vi "LVL device cluster to String.vi"(11 "Level Meter":T1) -> (3 "Data to send":string=":HEL:RES:ZERO:1.0:FULL:2.0:RES:PREP:MAG:3.0:TIM:4.0:PREP:PULS:MAG:5.0:TIM:6.0:DEL:7.0:PULS:HEL:NIT:FREQ:ZERO:8.0:FULL:9.0:FREQ:PPS:10.0:NIT")   [LabVIEW 2019, in "Mercury iXX.lvlib" / "Level Meter.lvlib"]
uses:
  Level Meter.lvlib
  Controls/Level Meter (Set).ctl
  Controls/Helium Configuration.ctl
  Controls/Resistance Configuration.ctl
  Controls/Pre-Pulse.ctl
  Controls/Pulse.ctl
  Controls/Nitrogen Configuration.ctl
  Controls/Frequency Configuration.ctl
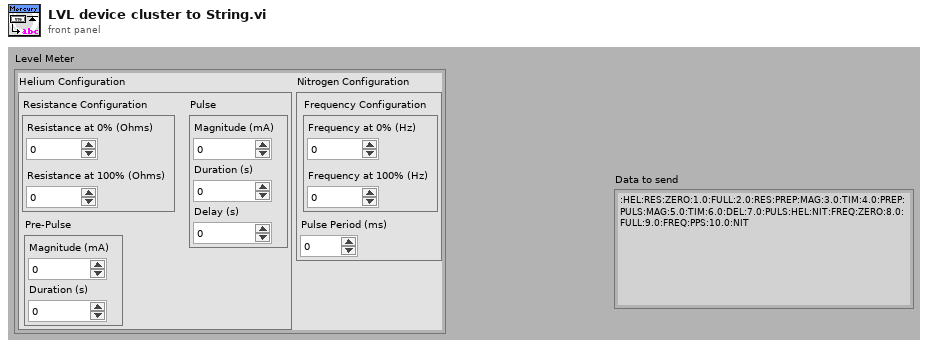
[diagram p1: front panel]
types:
  T1 = typedef "Mercury iXX.lvlib/Level Meter.lvlib/Level Meter (Set).ctl" = cluster{"Helium Configuration":T2, "Nitrogen Configuration":T6}
  T2 = typedef "Mercury iXX.lvlib/Level Meter.lvlib/Helium Configuration.ctl" = cluster{"Resistance Configuration":T3, "Pre-Pulse":T4, "Pulse":T5}
  T3 = typedef "Mercury iXX.lvlib/Level Meter.lvlib/Resistance Configuration.ctl" = cluster{"Res 0%":dbl, "Res 100%":dbl}
  T4 = typedef "Mercury iXX.lvlib/Level Meter.lvlib/Pre-Pulse.ctl" = cluster{"Magnitude":dbl, "Duration":dbl}
  T5 = typedef "Mercury iXX.lvlib/Level Meter.lvlib/Pulse.ctl" = cluster{"Magnitude":dbl, "Duration":dbl, "Delay":dbl}
  T6 = typedef "Mercury iXX.lvlib/Level Meter.lvlib/Nitrogen Configuration.ctl" = cluster{"Frequency Configuration":T7, "Pulse Period":dbl}
  T7 = typedef "Mercury iXX.lvlib/Level Meter.lvlib/Frequency Configuration.ctl" = cluster{"Freq 0%":dbl, "Freq 100%":dbl}
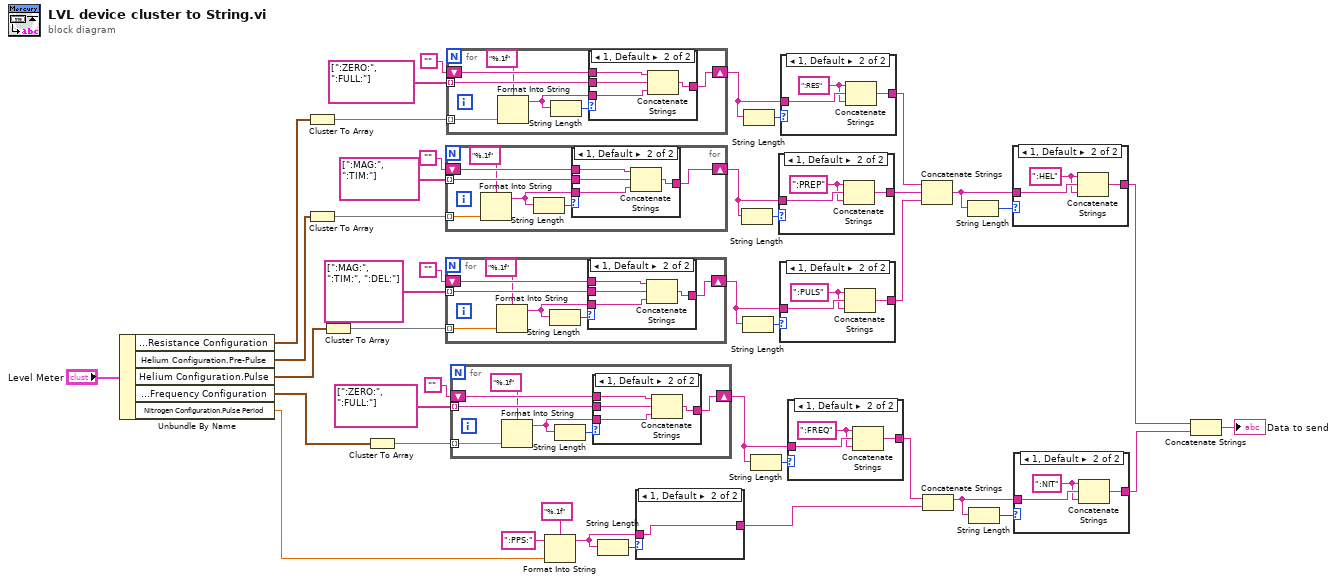
[diagram p0: block diagram]
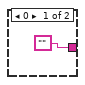
[diagram p2: hidden frame]
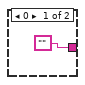
[diagram p3: hidden frame]
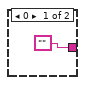
[diagram p4: hidden frame]
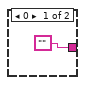
[diagram p5: hidden frame]
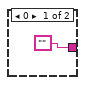
[diagram p6: hidden frame]
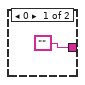
[diagram p7: hidden frame]
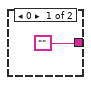
[diagram p10: hidden frame]
diagram:
  n1 = Unbundle By Name("Level Meter") -> ("Helium Configuration.Resistance Configuration"=w39:T3, "Helium Configuration.Pre-Pulse"=w34:T4, "Helium Configuration.Pulse"=w33:T5, "Nitrogen Configuration.Frequency Configuration"=w35:T7, "Nitrogen Configuration.Pulse Period"=w29:dbl)
  n2 = Cluster To Array(cluster=w39) -> (array=w27:dbl[])
  n3 = Cluster To Array(cluster=w34) -> (array=w25:dbl[])
  n4 = Cluster To Array(cluster=w33) -> (array=w19:dbl[])
  n5 = Cluster To Array(cluster=w35) -> (array=w36:dbl[])
  n6 = for {
    tunnel: w25 -> [w45] mode=indexing
    tunnel: string[] [":MAG:", ":TIM:"] ("Excitation") -> [w48] mode=indexing
    shift-right: [w47] -> w10
    shift-left: "" -> [w46]
    n7 = Format Into String(format string="%.1f", w45) -> (resulting string=w44:string)  [unwired: 2 in, 1 out]
    n8 = String Length(string=w44) -> (length=w49:i32)
    n9 = case shown="1, Default" w49 {
      tunnel: w44 -> [_ w53]
      tunnel: [w50 w54] -> w47
      tunnel: w48 -> [_ w52]
      tunnel: w46 -> [w50 w51]
      frame 0 {
      }
      frame 1, Default {
        n10 = Concatenate Strings(w51, w52, w53) -> (w54:string)
      }
    }
  }
  n11 = for {
    tunnel: w19 -> [w57] mode=indexing
    tunnel: string[] [":MAG:", ":TIM:", ":DEL:"] ("Excitation") -> [w60] mode=indexing
    shift-right: [w59] -> w13
    shift-left: "" -> [w58]
    n12 = Format Into String(format string="%.1f", w57) -> (resulting string=w56:string)  [unwired: 2 in, 1 out]
    n13 = String Length(string=w56) -> (length=w61:i32)
    n14 = case shown="1, Default" w61 {
      tunnel: w56 -> [_ w65]
      tunnel: [w62 w66] -> w59
      tunnel: w60 -> [_ w64]
      tunnel: w58 -> [w62 w63]
      frame 0 {
      }
      frame 1, Default {
        n15 = Concatenate Strings(w63, w64, w65) -> (w66:string)
      }
    }
  }
  n16 = for {
    tunnel: w27 -> [w69] mode=indexing
    tunnel: string[] [":ZERO:", ":FULL:"] ("Excitation") -> [w72] mode=indexing
    shift-right: [w71] -> w8
    shift-left: "" -> [w70]
    n17 = Format Into String(format string="%.1f", w69) -> (resulting string=w68:string)  [unwired: 2 in, 1 out]
    n18 = String Length(string=w68) -> (length=w73:i32)
    n19 = case shown="1, Default" w73 {
      tunnel: w68 -> [_ w77]
      tunnel: [w74 w78] -> w71
      tunnel: w72 -> [_ w76]
      tunnel: w70 -> [w74 w75]
      frame 0 {
      }
      frame 1, Default {
        n20 = Concatenate Strings(w75, w76, w77) -> (w78:string)
      }
    }
  }
  n21 = for {
    tunnel: w36 -> [w81] mode=indexing
    tunnel: string[] [":ZERO:", ":FULL:"] ("Excitation") -> [w84] mode=indexing
    shift-right: [w83] -> w17
    shift-left: "" -> [w82]
    n22 = Format Into String(format string="%.1f", w81) -> (resulting string=w80:string)  [unwired: 2 in, 1 out]
    n23 = String Length(string=w80) -> (length=w85:i32)
    n24 = case shown="1, Default" w85 {
      tunnel: w80 -> [_ w89]
      tunnel: [w86 w90] -> w83
      tunnel: w84 -> [_ w88]
      tunnel: w82 -> [w86 w87]
      frame 0 {
      }
      frame 1, Default {
        n25 = Concatenate Strings(w87, w88, w89) -> (w90:string)
      }
    }
  }
  n26 = Format Into String(format string="%.1f", initial string=":PPS:", w29) -> (resulting string=w31:string)  [unwired: 1 in, 1 out]
  n27 = String Length(string=w31) -> (length=w30:i32)
  n28 = case shown="1, Default" w30 {
    tunnel: w31 -> [_ w92]
    tunnel: ["" w92] -> w28
    frame 0 {
    }
    frame 1, Default {
    }
  }
  n29 = String Length(string=w10) -> (length=w11:i32)
  n30 = String Length(string=w13) -> (length=w14:i32)
  n31 = String Length(string=w8) -> (length=w9:i32)
  n32 = String Length(string=w17) -> (length=w18:i32)
  n33 = case shown="1, Default" w11 {
    tunnel: ["" w96] -> w6
    tunnel: w10 -> [_ w95]
    frame 0 {
    }
    frame 1, Default {
      w94 = ":PREP" ("string")
      n34 = Concatenate Strings(w94, w95, w94) -> (w96:string)
    }
  }
  n35 = case shown="1, Default" w14 {
    tunnel: ["" w100] -> w5
    tunnel: w13 -> [_ w99]
    frame 0 {
    }
    frame 1, Default {
      w98 = ":PULS" ("string")
      n36 = Concatenate Strings(w98, w99, w98) -> (w100:string)
    }
  }
  n37 = case shown="1, Default" w9 {
    tunnel: ["" w104] -> w7
    tunnel: w8 -> [_ w103]
    frame 0 {
    }
    frame 1, Default {
      w102 = ":RES" ("string")
      n38 = Concatenate Strings(w102, w103, w102) -> (w104:string)
    }
  }
  n39 = case shown="1, Default" w18 {
    tunnel: ["" w108] -> w16
    tunnel: w17 -> [_ w107]
    frame 0 {
    }
    frame 1, Default {
      w106 = ":FREQ" ("string")
      n40 = Concatenate Strings(w106, w107, w106) -> (w108:string)
    }
  }
  n41 = Concatenate Strings(w7, w6, w5) -> (w3:string)
  n42 = Concatenate Strings(w16, w28) -> (w22:string)
  n43 = String Length(string=w3) -> (length=w4:i32)
  n44 = String Length(string=w22) -> (length=w23:i32)
  n45 = case shown="1, Default" w4 {
    tunnel: ["" w112] -> w2
    tunnel: w3 -> [_ w111]
    frame 0 {
    }
    frame 1, Default {
      w110 = ":HEL" ("string")
      n46 = Concatenate Strings(w110, w111, w110) -> (w112:string)
    }
  }
  n47 = case shown="1, Default" w23 {
    tunnel: ["" w116] -> w21
    tunnel: w22 -> [_ w115]
    frame 0 {
    }
    frame 1, Default {
      w114 = ":NIT" ("string")
      n48 = Concatenate Strings(w114, w115, w114) -> (w116:string)
    }
  }
  n49 = Concatenate Strings(w2, w21) -> (→"Data to send":string)
